vi "Command with Logging.vi"(8 "error in (no error)":errorcluster, 10 "Event Details":T1, 11 "Instruments in":refnum<class "Instruments.lvclass">) -> (0 "error out":errorcluster, 3 "Instruments out":refnum<class "Instruments.lvclass">)   [LabVIEW 2023, in "Instruments.lvlib" / "Instruments.lvclass"]
uses:
  Library/Instruments.lvclass
  C:/Users/Public/Documents/Development/builds/Framework/Engine.lvlibp/Engine/Library/Engine.lvclass
  C:/Users/Public/Documents/Development/builds/Framework/Actor Framework.lvlibp/1abvi3w/vi.lib/ActorFramework/Actor/Actor.lvclass
  builds/Framework/Engine.lvlibp/Engine/Accessors/Read Report Q.vi
  builds/Framework/Actor Framework.lvlibp/1abvi3w/vi.lib/ActorFramework/Actor/Read Actor Label.vi
  builds/Tools/QDMH.lvlibp/Private/Enqueue Single Element.vi
  builds/Tools/QDMH.lvlibp/Library/QDMH.lvclass
  Library/Instruments.lvclass/Instruments.ctl
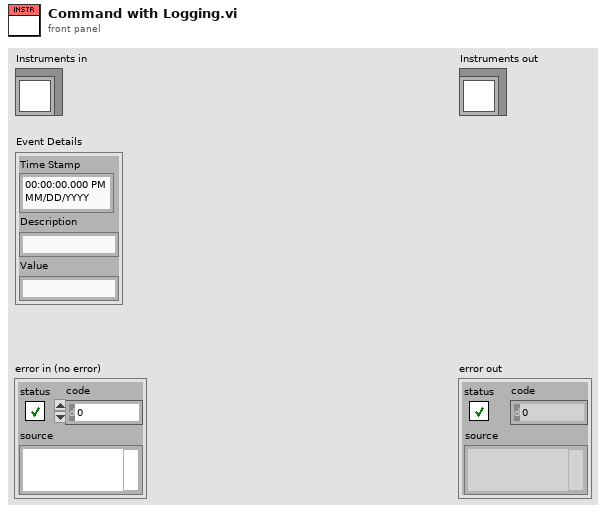
[diagram p1: front panel]
types:
  T1 = cluster{"Time Stamp":timestamp, "Description":string, "Value":string}
  T2 = cluster{"Time Stamp":timestamp, "Accessors:Actor Label":string, "Description":string, "Value":string}
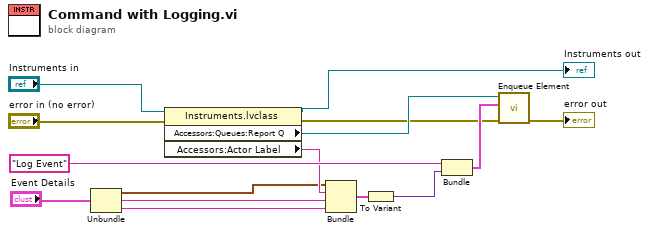
[diagram p0: block diagram]
diagram:
  n1 = Unbundle("Event Details") -> ("Time Stamp"=w6:timestamp, "Description"=w5:string, "Value"=w4:string)
  n2 = property class="Instruments.lvclass"(reference="Instruments in", error in="error in (no error)") -> (reference out=→"Instruments out":refnum<class "Instruments.lvclass">, error out=w3:errorcluster, "Accessors:Queues:Report Q"=w13:refnum<class "QDMH.lvclass">, "Accessors:Actor Label"=w7:string)
  n3 = Bundle("Time Stamp"=w6, "Accessors:Actor Label"=w7, "Description"=w5, "Value"=w4) -> (w8:T2)  [unwired: 1 in]
  n4 = To Variant(anything=w8) -> (Variant=w12:variant)
  n5 = Bundle("Log Event", "Variant"=w12) -> (w10:cluster{string, "Variant":variant})  [unwired: 1 in]
  n6 = call-poly "Enqueue Element.vi"("error in (no error)"=w3, "Message"=w10, "QDMH in"=w13) -> ("error out"=→"error out":errorcluster)  [unwired: 7 in, 1 out]
